vi "Page points.vi"(1 "Pages dimensions [ ]":T1[](array[typedef]), 2 "pageNum":i32=1) -> (0 "Page (points)":T1={"Start at page"=1, "Orientation"=enum."Portrait", "widht"=612.0, "height"=792.0, "Margin left"=72.0, "Margin right"=72.0, "Margin top"=72.0, "Margin bottom"=72.0})   [LabVIEW 2013]
doc: "Version 1.0\nDeveloped by Jean-Marc Simard\nCopyright © 2010, Exaprom Inc.\nAll rights reserved.\nLicense: BSD"
uses:
  Controls/Page dimensions.ctl
  Controls/Page Orientation.ctl
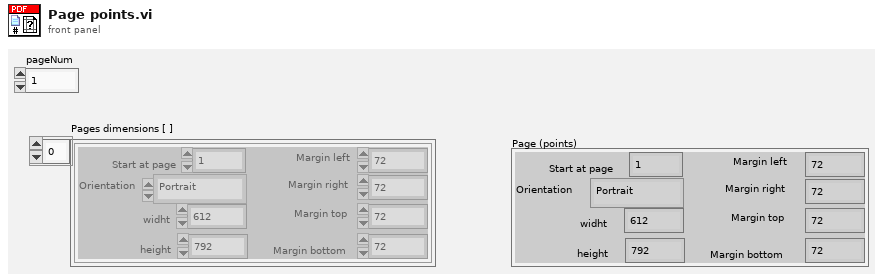
[diagram p1: front panel]
types:
  T1 = typedef "Page dimensions.ctl" = cluster{"Start at page":i32, "Orientation":T2, "widht":sgl, "height":sgl, "Margin left":sgl, "Margin right":sgl, "Margin top":sgl, "Margin bottom":sgl}
  T2 = typedef "Page Orientation.ctl" = enum16{"Portrait", "Landscape"}
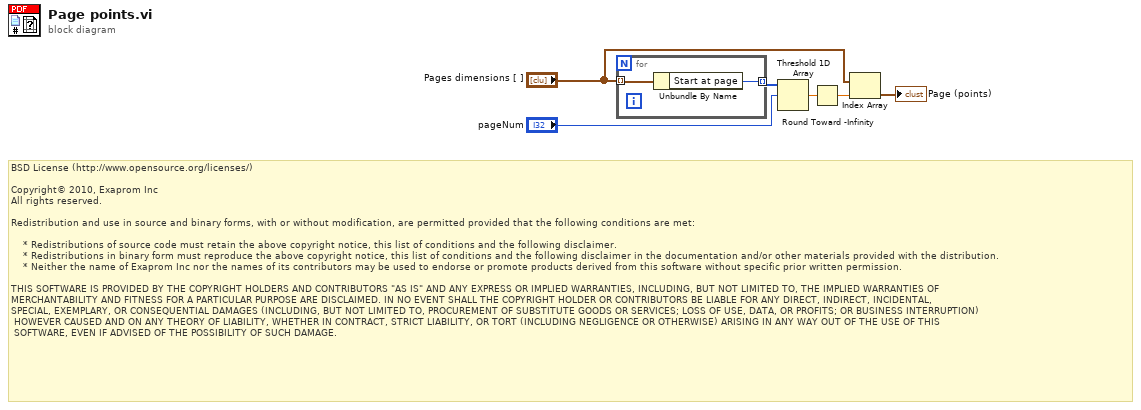
[diagram p0: block diagram]
diagram:
  # "BSD License (http://www.opensource.org/licenses/)\n\nCopyright© 2010, Exaprom Inc\nAll rights reserved.\n\nRedistribution and use in source and binary forms, with or without modification, are permitted provided that the following conditions are met:\n\n    * Redistributions of source code must retain the above copyright notice, this list of conditions and the following disclaimer.\n    * Redistributions in binary form must reproduce the above copyright notice, this list of conditions and the following disclaimer in the documentation and/or other materials provided with the distribution.\n    * Neither the name of Exaprom Inc nor the names of its contributors may be used to endorse or promote products derived from this software without specific prior written permission.\n\nTHIS SOFTWARE IS PROVIDED BY THE COPYRIGHT HOLDERS AND CONTRIBUTORS \"AS IS\" AND ANY EXPRESS OR IMPLIED WARRANTIES, INCLUDING, BUT NOT LIMITED TO, THE IMPLIED WARRANTIES OF \nMERCHANTABILITY AND FITNESS FOR A PARTICULAR PURPOSE ARE DISCLAIMED. IN NO EVENT SHALL THE COPYRIGHT HOLDER OR CONTRIBUTORS BE LIABLE FOR ANY DIRECT, INDIRECT, INCIDENTAL,\nSPECIAL, EXEMPLARY, OR CONSEQUENTIAL DAMAGES (INCLUDING, BUT NOT LIMITED TO, PROCUREMENT OF SUBSTITUTE GOODS OR SERVICES; LOSS OF USE, DATA, OR PROFITS; OR BUSINESS INTERRUPTION)\n HOWEVER CAUSED AND ON ANY THEORY OF LIABILITY, WHETHER IN CONTRACT, STRICT LIABILITY, OR TORT (INCLUDING NEGLIGENCE OR OTHERWISE) ARISING IN ANY WAY OUT OF THE USE OF THIS\n SOFTWARE, EVEN IF ADVISED OF THE POSSIBILITY OF SUCH DAMAGE."
  n1 = for {
    tunnel: "Pages dimensions [ ]" -> [w8] mode=indexing
    tunnel: [w7] -> w4 mode=indexing
    n2 = Unbundle By Name(w8) -> ("Start at page"=w7:i32)
  }
  n3 = Threshold 1D Array(2:"pageNum", 3:w4) -> (0:w5:dbl)  [unwired: 1 out]
  n4 = Round Toward -Infinity(1:w5) -> (0:w6:dbl)
  n5 = Index Array(array="Pages dimensions [ ]", index=w6) -> (element=→"Page (points)":T1)
